vi "Parse Token.vi"(10 "Token":enum8{"comment", "section", "key"}(ring), 11 "Line":string) -> (2 "Value":string, 3 "Name":string)   [LabVIEW 2022 SP3, in "LabVIEW-Config.lvlib"]
uses:
  LabVIEW-Config.lvlib
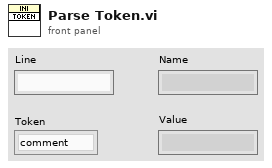
[diagram p1: front panel]
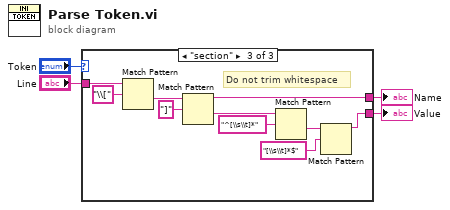
[diagram p0: block diagram]
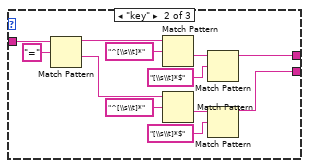
[diagram p3: hidden frame]
diagram:
  n1 = case shown="\"section\"" "Token" {
    tunnel: "Line" -> [w5 w12 w24]
    tunnel: [_ w11 w23] -> w2
    tunnel: [w5 w6 w18] -> w1
    frame "comment" {
    }
    frame "key" {
      n2 = Match Pattern(string=w12, regular expression="=") -> (before substring=w13:string, after substring=w7:string)  [unwired: 1 in, 2 out]
      n3 = Match Pattern(string=w13, regular expression="^[\\s\\t]*") -> (after substring=w16:string)  [unwired: 1 in, 3 out]
      n4 = Match Pattern(string=w7, regular expression="^[\\s\\t]*") -> (after substring=w8:string)  [unwired: 1 in, 3 out]
      n5 = Match Pattern(string=w16, regular expression="[\\s\\t]*$") -> (before substring=w11:string)  [unwired: 1 in, 3 out]
      n6 = Match Pattern(string=w8, regular expression="[\\s\\t]*$") -> (before substring=w6:string)  [unwired: 1 in, 3 out]
    }
    frame "section" {
      # "Do not trim whitespace"
      n7 = Match Pattern(string=w24, regular expression="\\[") -> (after substring=w25:string)  [unwired: 1 in, 3 out]
      n8 = Match Pattern(string=w25, regular expression="]") -> (before substring=w23:string, after substring=w19:string)  [unwired: 1 in, 2 out]
      n9 = Match Pattern(string=w19, regular expression="^[\\s\\t]*") -> (after substring=w20:string)  [unwired: 1 in, 3 out]
      n10 = Match Pattern(string=w20, regular expression="[\\s\\t]*$") -> (before substring=w18:string)  [unwired: 1 in, 3 out]
    }
  }
  "Value" <- w1
  "Name" <- w2
